vi "MVE Create Bound Variables.vi"(11 "Path":string) -> (0 "error out":errorcluster, 3 "cancelled":bool)   [LabVIEW 2016]
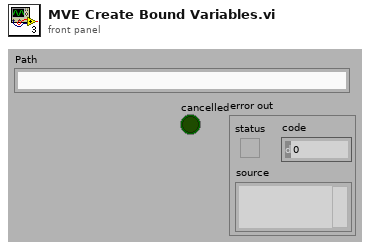
[diagram p1: front panel]
types:
  T1 = typedef "SCT Default Types.ctl" = cluster{"names":string[], "TDs":T2[]}
  T2 = typedef "NI_Variable.lvlib/Type Descriptor.ctl" = cluster{"Variant":variant}
  T3 = typedef "SCT Variable.ctl" = cluster{"Name":string, "TypeDesc":T2, "Type":string, "typedefs":string, "Attribs":T4, "FeaturePacks":string[], "Source":string}
  T4 = typedef "NI_Variable.lvlib/Attribs.ctl" = cluster{"Attrib":string, "Value":string}[]
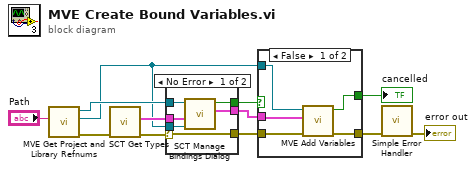
[diagram p0: block diagram]
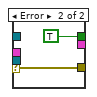
[diagram p2: hidden frame]
diagram:
  n1 = call <resource>:"MVE Get Project and Library Refnums.vi"("Full Path"="Path") -> ("error out"=w9:errorcluster, "ProjectItem Refnum"=w1:refnum<vi>, "Project Refnum"=w12:refnum<vi>)  [unwired: 8 in]
  n2 = call <resource>:"SCT Get Types.vi"("error in"=w9) -> ("error out"=w7:errorcluster, "default types"=w10:T1)  [unwired: 8 in, 1 out]
  n3 = case shown="No Error" w7 {
    selector: w7 -> [w18 w19]
    tunnel: w12 -> [w16 _]
    tunnel: w10 -> [w17 _]
    tunnel: [w15 TRUE ("Cancelled?")] -> w4
    tunnel: [w14 _] -> w8
    tunnel: [w18 w19] -> w6
    tunnel: w1 -> [w13 _]
    frame No Error {
      n4 = call <resource>:"SCT Manage Bindings Dialog.vi"("ParentItem Refnum"=w13, "default types"=w17, "Project Refnum"=w16) -> ("VariablesOut"=w14:T3[], "Cancelled?"=w15:bool)  [unwired: 6 in, 1 out]
    }
    frame Error {
    }
  }
  n5 = case shown="False" w4 {
    selector: w4 -> [_ w26]
    tunnel: w8 -> [w25 _]
    tunnel: w6 -> [w24 w27]
    tunnel: [w22 w27] -> w5
    tunnel: w1 -> [w23 _]
    tunnel: [w21 w26] -> w2
    frame False {
      n6 = call <resource>:"MVE Add Variables.vi"("error in (no error)"=w24, "variables"=w25, "ProjectItem Refnum"=w23) -> ("error out"=w22:errorcluster, "cancelled"=w21:bool)  [unwired: 7 in]
    }
    frame True {
    }
  }
  "cancelled" <- w2
  n7 = call <vilib>:"Simple Error Handler.vi"("error in (no error)"=w5) -> ("error out"=→"error out":errorcluster)  [unwired: 4 in, 4 out]
